vi "Sub_Get_Number_from_Remaining_Length.vi"(8 "error in (no error)":errorcluster, 10 "Remaining Length":u8[](array[numeric]) format="%x", 11 "connection ID":refnum<k5>) -> (0 "error out":errorcluster, 2 "X":u32, 3 "connection ID out":refnum<k5>)   [LabVIEW 2018, in "MQTT_Functions.lvlib"]
uses:
  MQTT_Functions.lvlib
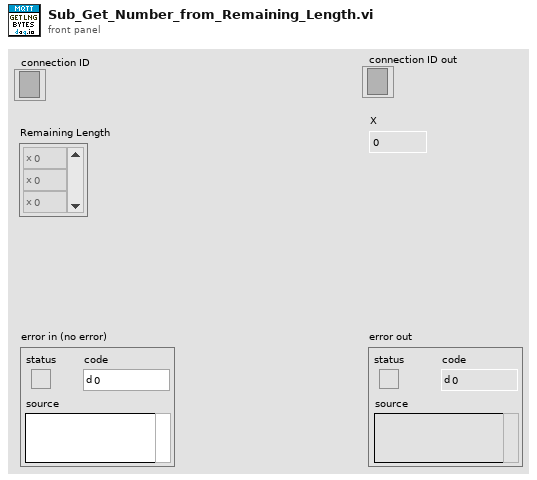
[diagram p1: front panel]
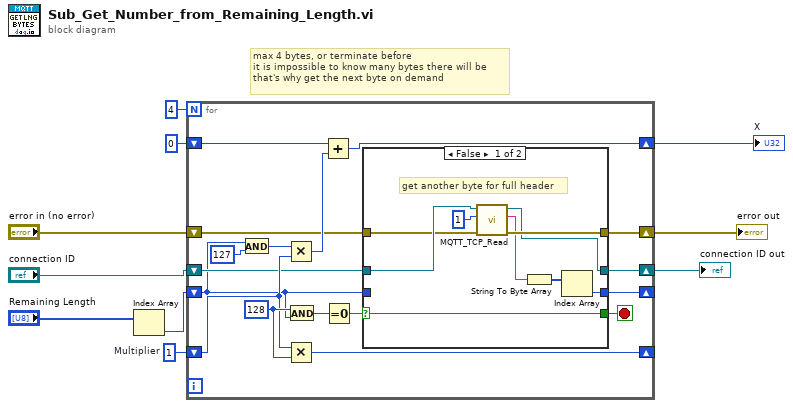
[diagram p0: block diagram]
diagram:
  w10 = u32 1  # Multiplier
  # "max 4 bytes, or terminate before\nit is impossible to know many bytes there will be\nthat's why get the next byte on demand"
  n1 = Index Array(array="Remaining Length") -> (element=w2:u8)  [unwired: 1 in]
  n2 = for {
    N: 4 -> [_]
    shift-right: [w27] -> _
    shift-left: w10 -> [w20]
    shift-right: [w22] -> w8
    shift-left: u32 0 -> [w24]
    shift-right: [w14] -> w4
    shift-left: "error in (no error)" -> [w15]
    shift-right: [w13] -> _
    shift-left: w2 -> [w12]
    shift-right: [w11] -> w1
    shift-left: "connection ID" -> [w16]
    stop <- w17 stop-if-true
    w21 = u32 128 ("y")
    n3 = And(x=w12, y=u8 127) -> (x .and. y?=w25:u8)
    n4 = Multiply(x=w25, y=w20) -> (x*y=w23:u32)
    n5 = Multiply(x=w20, y=w21) -> (x*y=w27:u32)
    n6 = And(x=w21, y=w12) -> (x .and. y?=w19:u32)
    n7 = Add(x=w24, y=w23) -> (x+y=w22:u32)
    n8 = Equal To 0?(x=w19) -> (x = 0?=w18:bool)
    n9 = case shown="False" w18 {
      selector: w18 -> [w36 w40]
      tunnel: [w36 w40] -> w17
      tunnel: w16 -> [w35 w37]
      tunnel: w15 -> [w33 w39]
      tunnel: [w32 w39] -> w14
      tunnel: [w29 w38] -> w13
      tunnel: w12 -> [_ w38]
      tunnel: [w28 w37] -> w11
      frame False {
        # "get another byte for full header"
        n10 = call "MQTT_TCP_Read.vi"("error in (no error)"=w33, "bytes to read"=1, "connection ID"=w35) -> ("error out"=w32:errorcluster, "data out"=w31:string, "connection ID out"=w28:refnum<k5>)  [unwired: 6 in]
        n11 = String To Byte Array(string=w31) -> (unsigned byte array=w30:u8[])
        n12 = Index Array(array=w30) -> (element=w29:u8)  [unwired: 1 in]
      }
      frame True {
      }
    }
  }
  "error out" <- w4
  "X" <- w8
  "connection ID out" <- w1
